vi "SeCrTs-Seq AO  Executer.vi"(8 "error in":errorcluster, 11 "Message Queue":refnum<queue>) -> (0 "error IO":errorcluster)   [LabVIEW 2022 SP3]
uses:
  <vilib>/Platform/TimedLoop/XDataNode/timing_clust.ctl
  <vilib>/Platform/TimedLoop/XDataNode/nitl_modes.ctl
  <vilib>/Platform/TimedLoop/XDataNode/wakeup.ctl
  68007add-2fa3-499d-ad7e-5bde15c16099.vi
  <vilib>/platform/TimedLoop/XDataNode/XDataNode.xnode
  <vilib>/Platform/TimedLoop/XDataNode/XDNodeRunTimeDep.lvlib
panel:
  out "x-y":u32
  out "Numeric 2":i32
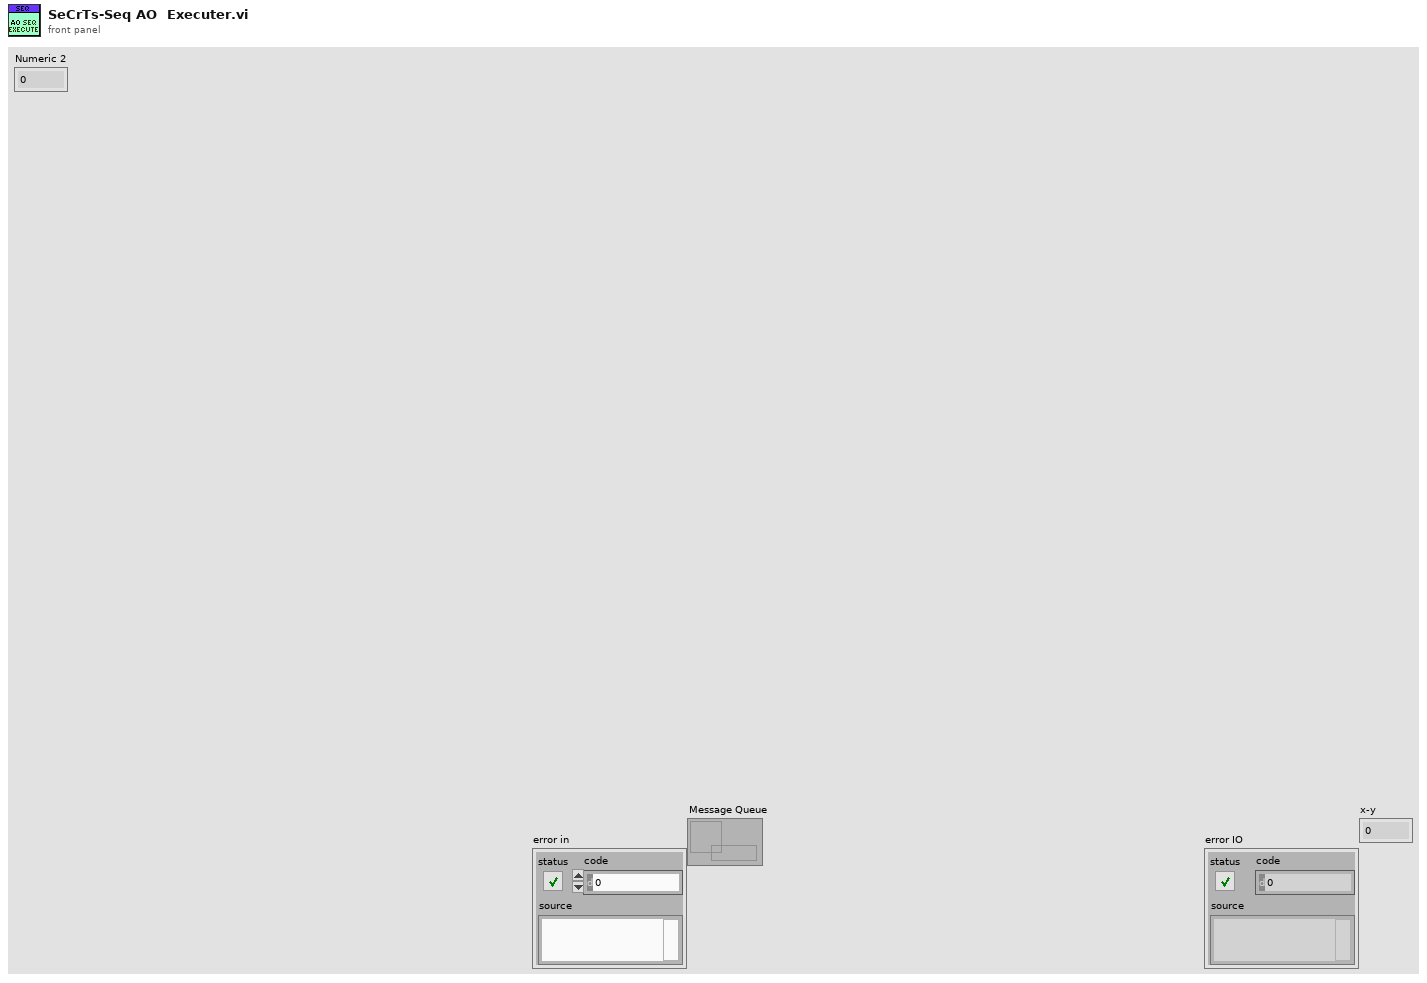
[diagram p1: front panel]
types:
  T1 = typedef "XDNodeRunTimeDep.lvlib/timing_clust.ctl" = cluster{"Expected End [f-1]":u64, "Actual End [f-1]":u64, "Finished Late? [f-1]":bool, "Expected End [i-1]":u64, "Actual End [i-1]":u64, "Finished Late? [i-1]":bool, "Expected Start [i]":u64, "Actual Start [i]":u64, "Expected Start [f]":u64, "Actual Start [f]":u64, "Source Name":string, "Structure Name":string, "Period":i64, "Deadline":i64, "Offset":i64, "Start":i64, "Priority":i32, "Timeout":i32, "Mode":T2, "Wakeup Reason":T3, "Error":errorcluster, "Source Type":string, "Secondary Source Type":string, "Global End Time":u64, "Global Start Time":u64, "Frame Duration":u64, "Iteration Duration":u64, "Assigned CPU":i32, "I/O Scan Engine Mode":u32}
  T2 = typedef "XDNodeRunTimeDep.lvlib/nitl_modes.ctl" = enum32{"No Change", "Process missed periods, maintain original phase", "Discard missed periods, maintain original phase", "Process missed periods, ignore original phase", "Discard missed periods, ignore original phase"}
  T3 = typedef "XDNodeRunTimeDep.lvlib/wakeup.ctl" = enum32{"Normal", "Aborted", "Asynchronous wakeup", "Timing source error", "Timed loop error", "Timeout"}
  T4 = enum16{"Init", "Read", "Write 'All'", "Write 'n'", "Write Safe Value", "Write Start Time", "Read 1"}
  T5 = cluster{"Manual HOLD":bool, "Automatic Hold AI":bool, "Abort":bool, "Automatic Hold DI":bool}
  T6 = cluster{"Start DAQ":bool, "Stop DAQ":bool, "RT Stop":bool, "RT Exit":bool, "Start Seq":bool}
  T7 = cluster{cluster{"Sr. No.":string, "Time CDT":string, "Component ID":string, "Data Type":string, "Condition":string, "Range/Position":string, "No of Samples for Pass":string, "Event Duration":string, "Continuous /Cumulative":string, "Expected Delay":string, "Failure case Seq":string, "Current Sequence":string}[]}[]
  T8 = cluster{"Sr. No.":string, "Time CDT":string, "Component ID":string, "Data Type":string, "Condition":string, "Range/Position":string, "No of Samples for Pass":string, "Event Duration":string, "Continuous /Cumulative":string, "Expected Delay":string, "Failure case Seq":string, "Current Sequence":string}[]
  T9 = cluster{"Sr. No.":string, "Time CDT":string, "Component ID":string, "Data Type":string, "Condition":string, "Range/Position":string, "No of Samples for Pass":string, "Event Duration":string, "Continuous /Cumulative":string, "Expected Delay":string, "Failure case Seq":string, "Current Sequence":string}
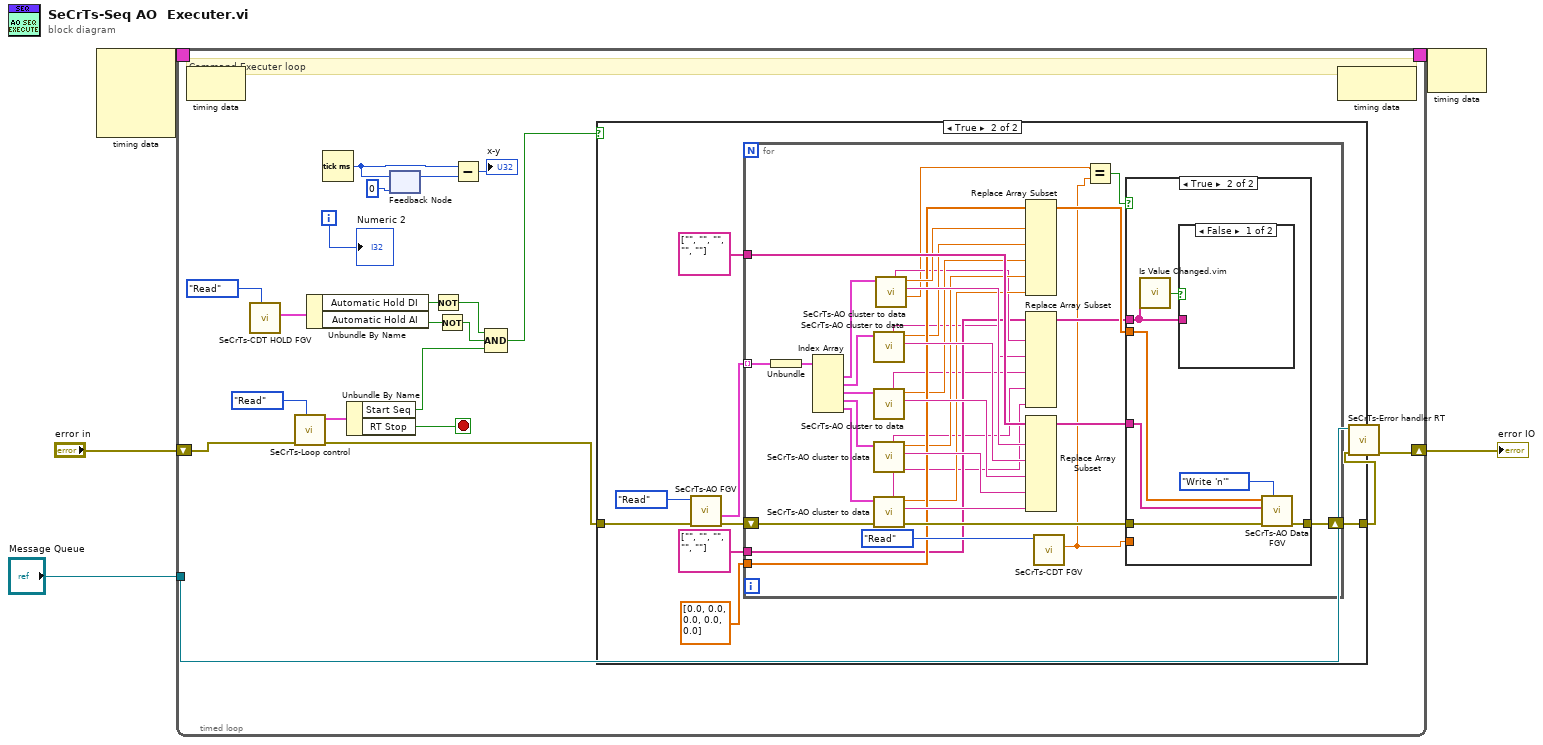
[diagram p0: block diagram]
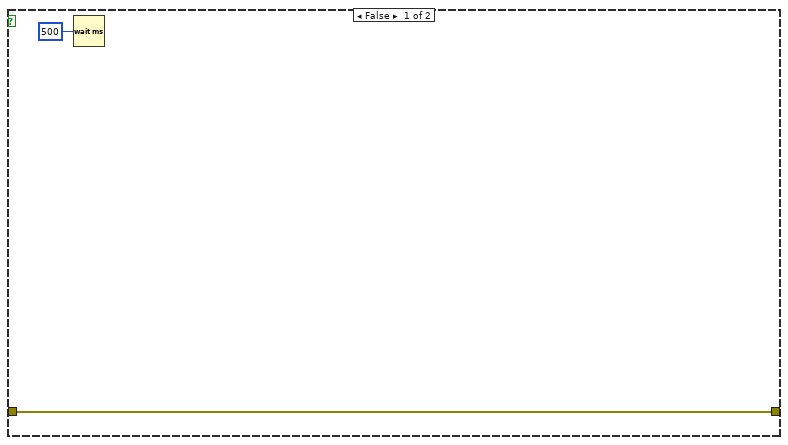
[diagram p2: hidden frame]
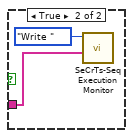
[diagram p4: hidden frame]
diagram:
  n1 = node-c288() -> (w3:T1)  [unwired: 4 in]
  n2 = timed-loop {
    shift-right: [w20] -> w5
    shift-left: "error in" -> [w11]
    timing: w3 -> [_]
    timing-out: [_] -> w2
    tunnel: "Message Queue" -> [w19]
    i -> [w26]
    stop <- w8 stop-if-true
    # "Command Executer loop"
    n3 = node-c288() -> ()  [unwired: 1 in, 1 out]
    n4 = call "SeCrTs-CDT HOLD FGV.vi"("Write/Read"=enum16{"Write", "Read"}."Read") -> ("HOLD and Abort Out"=w14:T5)  [unwired: 7 in, 1 out]
    n5 = call "SeCrTs-Loop control.vi"("Action"=enum16{"Init", "Write", "Read"}."Read", "error in (no error)"=w11) -> ("error Out"=w9:errorcluster, "Loop Control out"=w17:T6)  [unwired: 8 in]
    n6 = Unbundle By Name(w14) -> ("Automatic Hold DI"=w7:bool, "Automatic Hold AI"=w12:bool)
    n7 = Tick Count (ms)() -> (millisecond timer value=w24:u32)
    n8 = Unbundle By Name(w17) -> ("Start Seq"=w13:bool, "RT Stop"=w8:bool)
    n9 = feedback #1(u32 0 ("millisecond timer value")) -> (w25:u32)
    n10 = feedback-in #1(w24) -> ()
    n11 = Not(x=w7) -> (.not. x?=w6:bool)
    n12 = Not(x=w12) -> (.not. x?=w15:bool)
    n13 = Subtract(x=w24, y=w25) -> (x-y=→"x-y":u32)
    n14 = Compound Arithmetic op=AND(w6, w15, w13) -> (w10:bool)
    n15 = case shown="True" w10 {
      tunnel: w9 -> [w29 w34]
      tunnel: [w29 w38] -> w21
      frame False {
        n16 = Wait (ms)(milliseconds to wait=u32 500) -> ()  [unwired: 1 out]
      }
      frame True {
        n17 = call "SeCrTs-AO FGV.vi"("error in"=w34, "Enum"=enum16{"Read", "Write "}."Read") -> ("error out"=w33:errorcluster, "AO Seq  OUT"=w32:T7)  [unwired: 8 in]
        n18 = for {
          tunnel: w32 -> [w72] mode=indexing
          tunnel: string[] ["", "", "", "", ""] ("appended array") -> [w62]
          tunnel: dbl[] [0.0, 0.0, 0.0, 0.0, 0.0] ("appended array") -> [w55]
          shift-right: [w63] -> w38
          shift-left: w33 -> [w64]
          tunnel: string[] ["", "", "", "", ""] ("appended array") -> [w47]
          n19 = Unbundle(w72) -> (w71:T8)
          n20 = Index Array(array=w71) -> (element #1=w70:T9, element #2=w69:T9, element #3=w68:T9, element #4=w67:T9, element #5=w66:T9)  [unwired: 5 in]
          n21 = call "SeCrTs-AO cluster to data .vi"("output cluster"=w69) -> ("Component ID"=w60:string, "Value"=w54:dbl, "concatenated string"=w46:string)  [unwired: 7 in, 1 out]
          n22 = call "SeCrTs-AO cluster to data .vi"("output cluster"=w68) -> ("Component ID"=w59:string, "Value"=w53:dbl, "concatenated string"=w45:string)  [unwired: 7 in, 1 out]
          n23 = call "SeCrTs-AO cluster to data .vi"("output cluster"=w67) -> ("Component ID"=w58:string, "Value"=w52:dbl, "concatenated string"=w44:string)  [unwired: 7 in, 1 out]
          n24 = call "SeCrTs-AO cluster to data .vi"("output cluster"=w66) -> ("Component ID"=w57:string, "Value"=w51:dbl, "concatenated string"=w43:string)  [unwired: 7 in, 1 out]
          n25 = call "SeCrTs-AO cluster to data .vi"("output cluster"=w70) -> ("Numeric"=w41:dbl, "Component ID"=w61:string, "Value"=w56:dbl, "concatenated string"=w48:string)  [unwired: 7 in]
          n26 = Replace Array Subset(array=w55, new element #1=w56, new element #2=w54, new element #3=w53, new element #4=w52, new element #5=w51) -> (w50:dbl[])  [unwired: 5 in]
          n27 = Replace Array Subset(array=w47, new element #1=w48, new element #2=w46, new element #3=w45, new element #4=w44, new element #5=w43) -> (w42:string[])  [unwired: 5 in]
          n28 = Replace Array Subset(array=w62, new element #1=w61, new element #2=w60, new element #3=w59, new element #4=w58, new element #5=w57) -> (w49:string[])  [unwired: 5 in]
          n29 = call "SeCrTs-CDT FGV.vi"("Write/Read"=enum16{"Write", "Read"}."Read") -> ("CDT Out"=w40:dbl)  [unwired: 9 in, 1 out]
          n30 = Equal?(x=w41, y=w40) -> (x = y?=w39:bool)
          n31 = case shown="True" w39 {
            tunnel: w64 -> [w73 w80]
            tunnel: [w73 w79] -> w63
            tunnel: w40 -> [_ _]
            tunnel: w50 -> [_ w78]
            tunnel: w49 -> [_ w77]
            tunnel: w42 -> [_ w74]
            frame False {
            }
            frame True {
              n32 = call "Is Value Changed.vim"("value"=w74) -> ("changed or first call?"=w75:bool)
              n33 = case shown="False" w75 {
                tunnel: w74 -> [_ w81]
                frame False {
                }
                frame True {
                  n34 = call "SeCrTs-Seq Execution Monitor.vi"("Seq Monitor"=w81, "Enum"=enum16{"Read", "Write "}."Write ") -> ()  [unwired: 8 in, 2 out]
                }
              }
              n35 = call "SeCrTs-AO Data FGV.vi"("Option"=T4."Write 'n'", "error in (no error)"=w80, "AO Channel Names"=w77, "AO Values In"=w78) -> ("error out"=w79:errorcluster)  [unwired: 3 in, 4 out]
            }
          }
        }
      }
    }
    n36 = node-c288() -> ()  [unwired: 1 in, 1 out]
    n37 = call "SeCrTs-Error handler RT.vi"("error in"=w21, "Message Queue"=w19) -> ("error out"=w20:errorcluster)  [unwired: 8 in, 1 out]
    "Numeric 2" <- w26
  }
  "error IO" <- w5
  n38 = node-c288(w2) -> ()  [unwired: 1 out]
